vi "_Check_If_Error.vi"(8 "error in (no error)":errorcluster, 11 "Postgres Connector In":refnum<class "Postgres Connector.lvclass">) -> (0 "error out":errorcluster, 3 "Postgres Connector Out":refnum<class "Postgres Connector.lvclass">)   [LabVIEW 2020, in "Postgres Connector.lvclass"]
uses:
  Postgres Connector.lvclass
  Cluster_Reader_Infos.ctl
  Enum_RowDescription_State_Machine.ctl
  Postgres Connector.lvclass/Postgres Connector.ctl
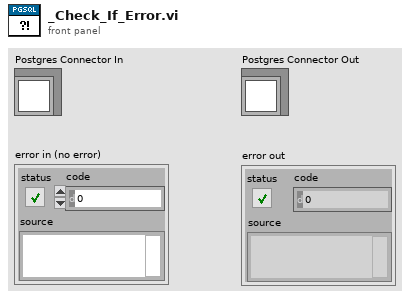
[diagram p1: front panel]
types:
  T1 = typedef "Postgres Connector.lvclass/Enum_RowDescription_State_Machine.ctl" = enum16{"Check For Error", "Wait For T", "Wait For D", "Wait For Z", "C Byte Length", "Z Byte Length", "n Byte Length", "Byte Length", "Get Infos", "Check For End", "Flush", "Quit"}
  T2 = typedef "Postgres Connector.lvclass/Cluster_Reader_Infos.ctl" = cluster{"Byte Length":i32}
  T3 = enum16{"Standard", "Buffered", "CRLF", "Immediate"}
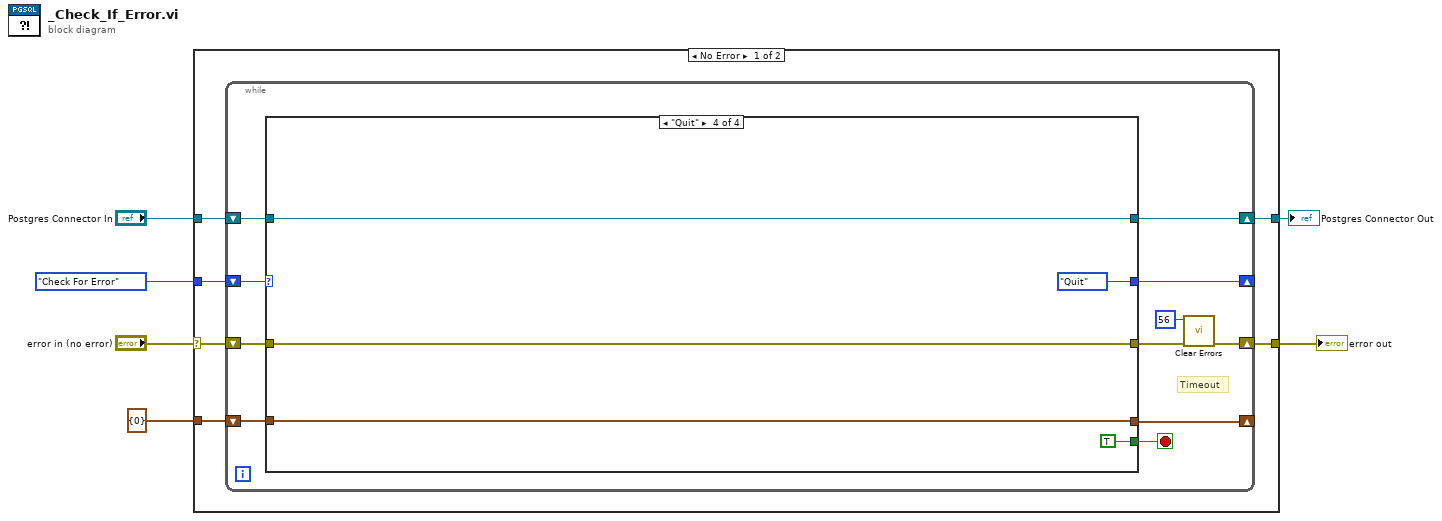
[diagram p0: block diagram]
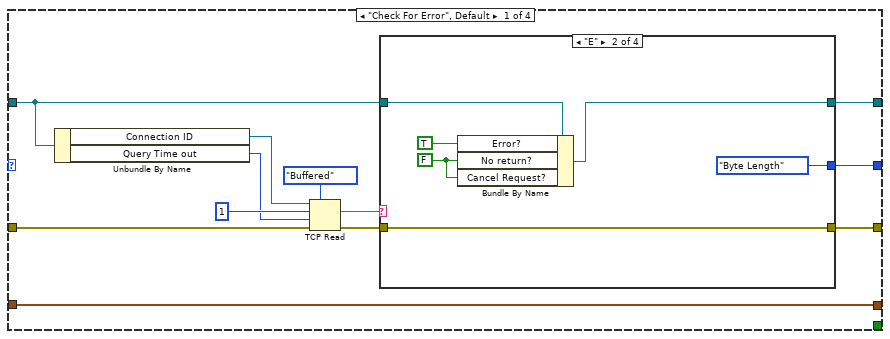
[diagram p2: hidden frame]
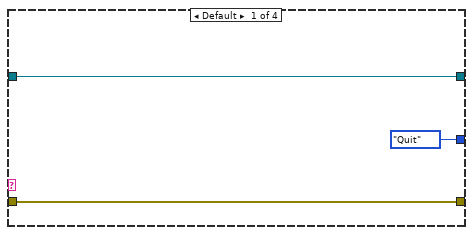
[diagram p3: hidden frame]
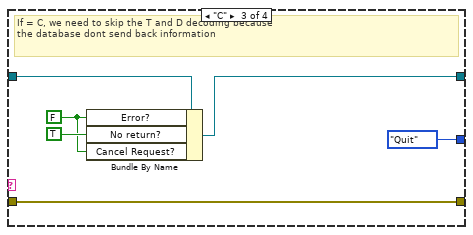
[diagram p4: hidden frame]
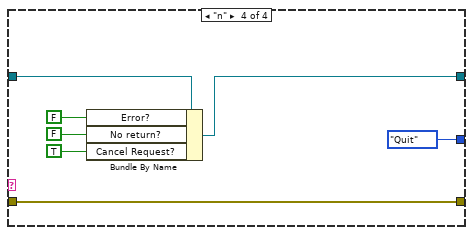
[diagram p5: hidden frame]
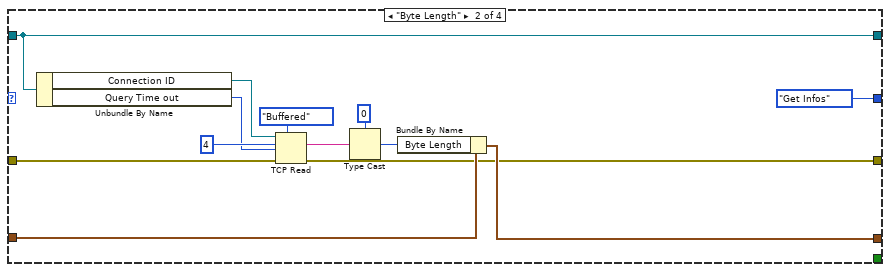
[diagram p6: hidden frame]
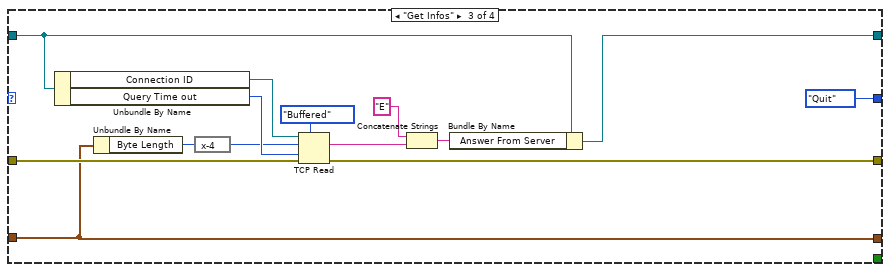
[diagram p7: hidden frame]
diagram:
  n1 = case shown="No Error" "error in (no error)" {
    selector: "error in (no error)" -> [w12 w91]
    tunnel: "Postgres Connector In" -> [w7 w90]
    tunnel: Enum_RowDescription_State_Machine."Check For Error" -> [w11 _]
    tunnel: [w10 w91] -> w4
    tunnel: T2 {"Byte Length"=0} ("Reader_Infos") -> [w9 _]
    tunnel: [w8 w90] -> w1
    frame No Error {
      n2 = while {
        shift-right: [w20] -> w10
        shift-left: w12 -> [w23]
        shift-right: [w18] -> _
        shift-left: w11 -> [w22]
        shift-right: [w16] -> _
        shift-left: w9 -> [w17]
        shift-right: [w14] -> w8
        shift-left: w7 -> [w13]
        stop <- w15 stop-if-true
        # "Timeout"
        n3 = case shown="\"Quit\"" w22 {
          tunnel: w23 -> [w32 w64 w83 w88]
          tunnel: [w24 w61 w82 w88] -> w21
          tunnel: [w25 Enum_RowDescription_State_Machine."Get Infos" Enum_RowDescription_State_Machine."Quit" Enum_RowDescription_State_Machine."Quit"] -> w18
          tunnel: w17 -> [w31 w63 w80 w89]
          tunnel: [w31 w62 w80 w89] -> w16
          tunnel: [_ _ _ TRUE] -> w15
          tunnel: [w26 w59 w77 w85] -> w14
          tunnel: w13 -> [w27 w59 w78 w85]
          frame "Check For Error", Default {
            n4 = Unbundle By Name(w27) -> ("Connection ID"=w34:refnum<k5>, "Query Time out"=w30:i32)
            n5 = TCP Read(connection ID=w34, bytes to read=1, error in (no error)=w32, 7:T3."Buffered" ("mode (standard)"), 9:w30) -> (data out=w28:string, error out=w29:errorcluster)  [unwired: 1 out]
            n6 = case shown="\"E\"" w28 {
              tunnel: w29 -> [w36 w39 w46 w53]
              tunnel: w27 -> [w38 w44 w50 w57]
              tunnel: [w38 w42 w49 w56] -> w26
              tunnel: [Enum_RowDescription_State_Machine."Quit" Enum_RowDescription_State_Machine."Byte Length" Enum_RowDescription_State_Machine."Quit" Enum_RowDescription_State_Machine."Quit"] -> w25
              tunnel: [w36 w39 w46 w53] -> w24
              frame Default {
              }
              frame "E" {
                w40 = FALSE ("No return?")
                n7 = Bundle By Name(cluster=w44, "Error?"=TRUE, "No return?"=w40, "Cancel Request?"=w40) -> (w42:refnum<class "Postgres Connector.lvclass">)
              }
              frame "C" {
                w45 = FALSE ("Error?")
                # "If = C, we need to skip the T and D decoding because \nthe database dont send back information"
                n8 = Bundle By Name(cluster=w50, "Error?"=w45, "No return?"=TRUE, "Cancel Request?"=w45) -> (w49:refnum<class "Postgres Connector.lvclass">)
              }
              frame "n" {
                n9 = Bundle By Name(cluster=w57, "Error?"=FALSE, "No return?"=FALSE, "Cancel Request?"=TRUE) -> (w56:refnum<class "Postgres Connector.lvclass">)
              }
            }
          }
          frame "Byte Length" {
            n10 = Unbundle By Name(w59) -> ("Connection ID"=w70:refnum<k5>, "Query Time out"=w58:i32)
            n11 = TCP Read(connection ID=w70, bytes to read=4, error in (no error)=w64, 7:T3."Buffered" ("mode (standard)"), 9:w58) -> (data out=w69:string, error out=w61:errorcluster)  [unwired: 1 out]
            n12 = Type Cast(type=0, x=w69) -> (*(type *) &x=w68:i32)
            n13 = Bundle By Name(cluster=w63, "Byte Length"=w68) -> (w62:T2)
          }
          frame "Get Infos" {
            n14 = Unbundle By Name(w78) -> ("Connection ID"=w79:refnum<k5>, "Query Time out"=w73:i32)
            n15 = Unbundle By Name(w80) -> ("Byte Length"=w72:i32)
            n16 = expression code="x-4"(w72) -> (w71:i32)
            n17 = TCP Read(connection ID=w79, bytes to read=w71, error in (no error)=w83, 7:T3."Buffered" ("mode (standard)"), 9:w73) -> (data out=w76:string, error out=w82:errorcluster)  [unwired: 1 out]
            n18 = Concatenate Strings("E" ("string"), w76) -> (w75:string)
            n19 = Bundle By Name(cluster=w78, "Answer From Server"=w75) -> (w77:refnum<class "Postgres Connector.lvclass">)
          }
          frame "Quit" {
          }
        }
        n20 = call <vilib>:"Clear Errors.vi"("error in (no error)"=w21, "specific error code to clear (0: all)"=56) -> ("error out"=w20:errorcluster)  [unwired: 4 in, 1 out]
      }
    }
    frame Error {
    }
  }
  "error out" <- w4
  "Postgres Connector Out" <- w1
